vi "CheckPiecesToScore-C.vi"(11 "Params":string[][](array[string])) -> ()   [LabVIEW 2018]
uses:
  Framework/Robot Global Data.vi
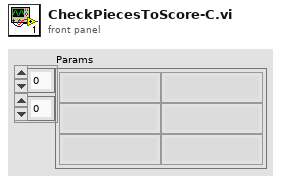
[diagram p1: front panel]
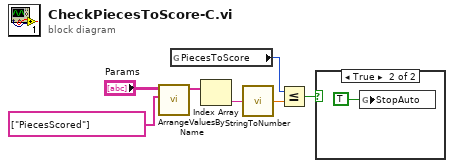
[diagram p0: block diagram]
diagram:
  n1 = call "ArrangeValuesByName.vi"("Names"=string[] ["PiecesScored"], "Names/Values in"="Params") -> ("Values Out"=w2:string[])  [unwired: 9 in]
  n2 = global read "Robot Global Data.vi" "PiecesToScore"() -> (w7:u16)
  n3 = Index Array(array=w2) -> (element=w1:string)  [unwired: 1 in]
  n4 = call "StringToNumber.vi"("String"=w1) -> ("Output"=w6:dbl)
  n5 = Less Or Equal?(x=w7, y=w6) -> (x <= y?=w5:bool)
  n6 = case shown="True" w5 {
    frame False {
    }
    frame True {
      n7 = global write "Robot Global Data.vi" "StopAuto"(TRUE ("StopAuto")) -> ()
    }
  }
